vi "Box.vi"(10 "data":i32) -> (2 "CustomeNode out":refnum<class "CustomeNode.lvclass">)   [LabVIEW 2021, in "CustomeNode.lvclass"]
uses:
  CustomeNode.lvclass
  CustomeNode.lvclass/CustomeNode.ctl
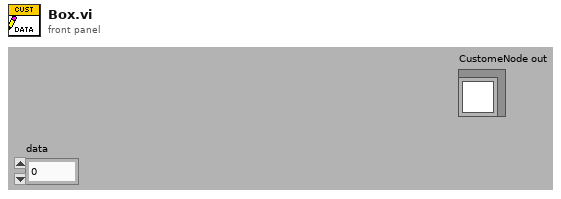
[diagram p1: front panel]
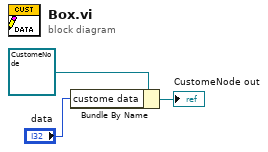
[diagram p0: block diagram]
diagram:
  n1 = Bundle By Name(cluster=refnum<class "CustomeNode.lvclass"> refnum ("CustomeNode in"), "custome data"="data") -> (→"CustomeNode out":refnum<class "CustomeNode.lvclass">)
